vi "Delete from Storage.vi"(8 "error in (no error)":errorcluster, 10 "Key":string="myhome/kitchen/temp", 11 "Zenoh in":refnum<class "Zenoh.lvclass">) -> (0 "error out":errorcluster)   [LabVIEW 2021, in "Zenoh.lvclass"]
doc: "Remove the key from any storage elements on the system."
uses:
  Zenoh.lvclass
  Zenoh.lvclass/Zenoh.ctl
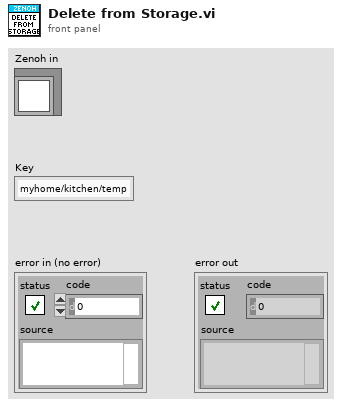
[diagram p1: front panel]
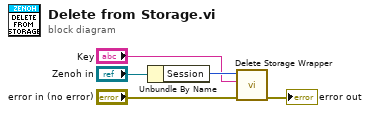
[diagram p0: block diagram]
diagram:
  n1 = Unbundle By Name("Zenoh in") -> ("Session"=w3:u64)
  n2 = call "Delete Storage Wrapper.vi"("error in (no error)"="error in (no error)", "key"="Key", "Session in"=w3) -> ("error out"=→"error out":errorcluster)  [unwired: 8 in]
